vi "GA_Plot.vi"(8 "max index(es)":i32, 10 "pop(500*20)":i32[][](array[numeric]), 11 "reference":refnum<vi>) -> ()   [LabVIEW 2018]
uses:
  GA_Global.vi
panel:
  out "subarray":i32[](array[numeric])
  in  "XY Graph":cluster{dbl[], dbl[]}[](graph)
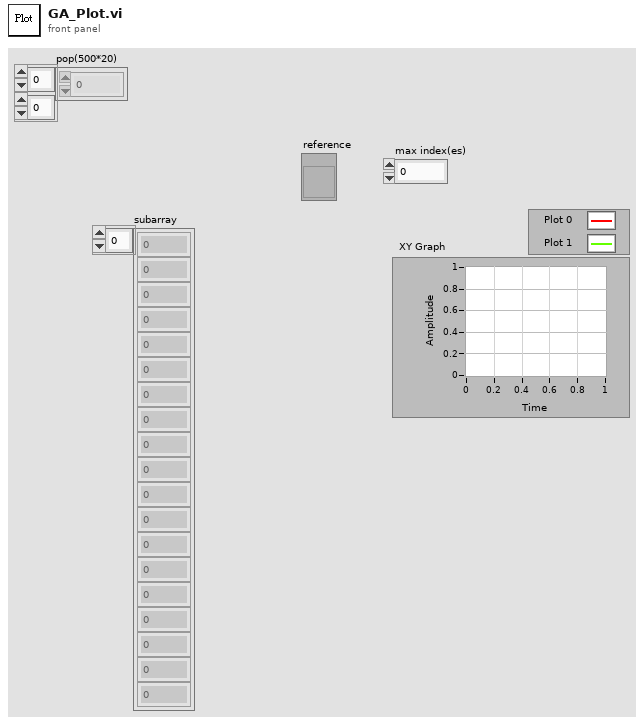
[diagram p1: front panel]
types:
  T1 = cluster{"city_position(20*2)":dbl[], "city_position(20*2)":dbl[]}
  T2 = cluster{"city_position(20*2)":dbl[], "city_position(20*2)":dbl[]}[]
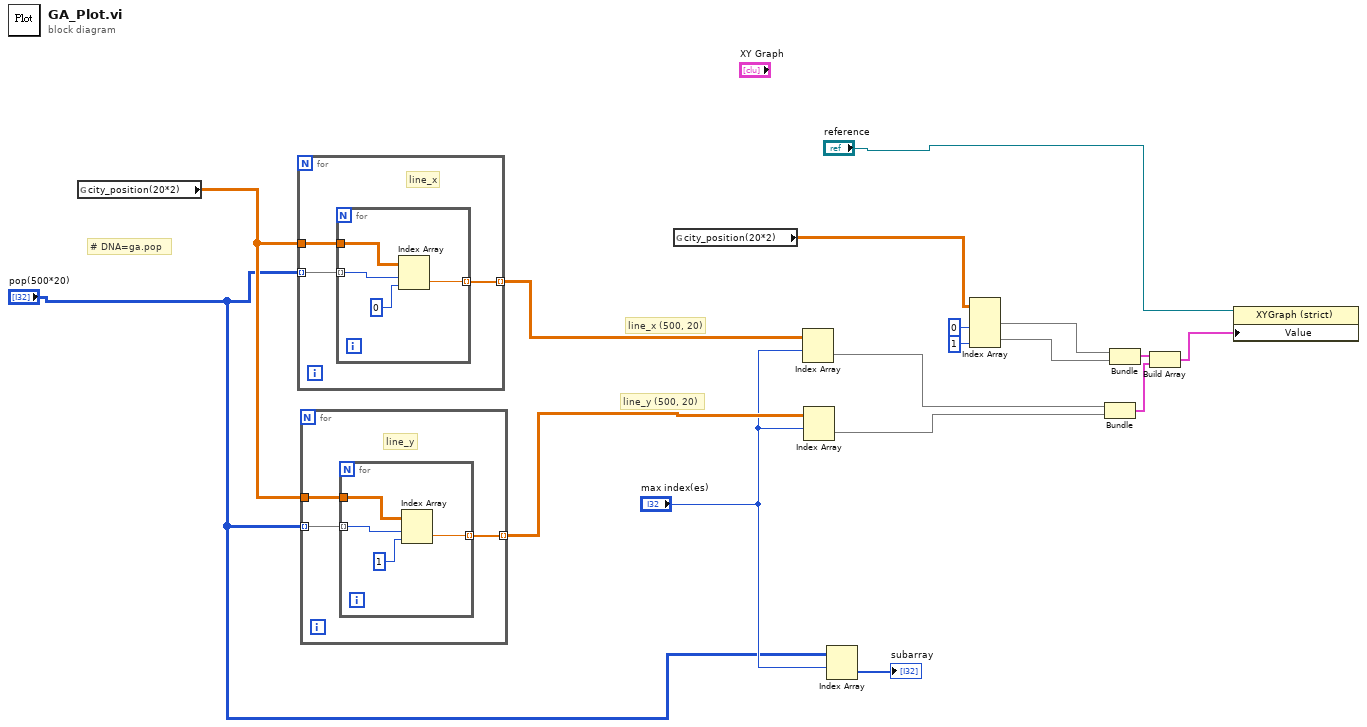
[diagram p0: block diagram]
diagram:
  # "line_y (500, 20)"
  # "line_x (500, 20)"
  # "# DNA=ga.pop"
  n1 = global read "GA_Global.vi" "city_position(20*2)"() -> (w6:dbl[][])
  n2 = for {
    tunnel: w6 -> [w20]
    tunnel: "pop(500*20)" -> [w19] mode=indexing
    tunnel: [w18] -> w5 mode=indexing
    # "line_x"
    n3 = for {
      tunnel: w20 -> [w24]
      tunnel: w19 -> [w23] mode=indexing
      tunnel: [w21] -> w18 mode=indexing
      n4 = Index Array(array=w24, index (row)=w23, index (col)=0 ("disabled index (col)")) -> (element=w21:dbl)
    }
  }
  n5 = for {
    tunnel: w6 -> [w27]
    tunnel: "pop(500*20)" -> [w26] mode=indexing
    tunnel: [w25] -> w4 mode=indexing
    # "line_y"
    n6 = for {
      tunnel: w27 -> [w31]
      tunnel: w26 -> [w30] mode=indexing
      tunnel: [w28] -> w25 mode=indexing
      n7 = Index Array(array=w31, index (row)=w30, index (col)=1 ("disabled index (col)")) -> (element=w28:dbl)
    }
  }
  n8 = global read "GA_Global.vi" "city_position(20*2)"() -> (w11:dbl[][])
  n9 = Index Array(array=w5, index (row)="max index(es)") -> (element=w8:dbl[])  [unwired: 1 in]
  n10 = Index Array(array=w4, index (row)="max index(es)") -> (element=w7:dbl[])  [unwired: 1 in]
  n11 = Index Array(array="pop(500*20)", index (row)="max index(es)") -> (element=→"subarray":i32[])  [unwired: 1 in]
  n12 = Index Array "Index Array"(array=w11, index (col) #1=0 ("disabled index (col)"), index (col) #2=1 ("index (col)")) -> (element #1=w17:dbl[], element #2=w14:dbl[])  [unwired: 2 in]
  n13 = Bundle(w8, w7) -> (w9:cluster{dbl[], dbl[]})  [unwired: 1 in]
  n14 = Bundle("city_position(20*2)"=w17, "city_position(20*2)"=w14) -> (w13:T1)  [unwired: 1 in]
  n15 = Build Array(w13, w9) -> (w12:T2)
  n16 = property class="XYGraph (strict)"(reference="reference", "Value"=w12) -> ()  [unwired: 1 in, 2 out]
